vi "Vision 통합 수정필요.vi"() -> ()   [LabVIEW 2016]
uses:
  <vilib>/vision/Classification.llb/IMAQ Classifier Nearest Neighbor options.ctl
  <vilib>/vision/NI_Vision_Development_Module.lvlib
  <vilib>/ptbypt/NI_PtbyPt.lvlib
panel:
  in  "경로 설정":enum32{"주차", "유턴", "곡선", "동적"}(tab)
  in  "File Path (Particle Classification 1)":path=path "C:/Users/SeongHyeon/Desktop/[Github]_GPS Team/labview_program/작업중인 모든 Vi, dll파일 모음/전체프로그램/Sub Vi/Sensor/Vision Reference/주차.clf"
  in  "유턴File Path":path=path "C:/Users/SeongHyeon/Desktop/[Github]_GPS Team/labview_program/작업중인 모든 Vi, dll파일 모음/전체프로그램/Sub Vi/Sensor/Vision Reference/유턴2.clf"
  in  "곡선File Path 2":path=path "C:/Users/SeongHyeon/Desktop/[Github]_GPS Team/labview_program/작업중인 모든 Vi, dll파일 모음/전체프로그램/Sub Vi/Sensor/Vision Reference/곡선2.clf"
  in  "동적장애물File Path 4":path=path "C:/Users/SeongHyeon/Desktop/[Github]_GPS Team/labview_program/작업중인 모든 Vi, dll파일 모음/전체프로그램/Sub Vi/Sensor/Vision Reference/동적 장애물 Dark.clf"
  in  "Parameter 설정":enum32{"주차", "유턴", "곡선", "동적"}(tab)
  in  "주차 Paramaters":T2={"Preprocessing Options"={"Method"=-1, "Looking for"=1, "Threshold Range"={"Lower value"=0.0, "Upper value"=0.0}, "Threshold Limits"={"Lower value"=0.0, "Upper value"=0.0}, "Reject Border"=FALSE, "# of Erosions"=0, "Kernel Size"={"Lower value"=0, "Upper value"=0}, "Deviation Factor"=0.0}, "Nearest Neighbor Options"={"Method"=0, "Metric"=0, "k"=0}, "Particle Options"={"Scale Dependant"=FALSE, "Scale Factor"=0.0, "Symmetry Dependant"=FALSE, "Symmetry Factor"=0.0}} {"Preprocessing Options"."Deviation Factor" min=0.0; "Preprocessing Options"."Threshold Limits"."Upper value" format="%.2f"; "Preprocessing Options"."Threshold Limits"."Lower value" format="%.2f"; "Preprocessing Options"."Threshold Range"."Upper value" format="%.2f"; "Preprocessing Options"."Threshold Range"."Lower value" format="%.2f"; "Preprocessing Options"."# of Erosions" min=0; "Preprocessing Options"."Method" items=["Manual Threshold"=-1, "-"=-2, "Auto Threshold: Clustering"=0, "Auto Threshold: Entropy"=1, "Auto Threshold: Metric"=2, "Auto Threshold: Moments"=3, "Auto Threshold: Inter-class Variance"=4, "--"=-3, "Local Threshold: Niblack"=5, "Local Threshold: BG Correction"=6]; "Preprocessing Options"."Looking for" items=["Bright Objects", "Dark Objects"]; "Nearest Neighbor Options"."Method" items=["Nearest Neighbor", "K Nearest Neighbor", "Minimum Mean Distance"]; "Nearest Neighbor Options"."Metric" items=["Maximum", "Sum", "Euclidean"]; "Nearest Neighbor Options"."k" min=3}
  in  "유턴 Paramaters":T2={"Preprocessing Options"={"Method"=-1, "Looking for"=1, "Threshold Range"={"Lower value"=0.0, "Upper value"=0.0}, "Threshold Limits"={"Lower value"=0.0, "Upper value"=0.0}, "Reject Border"=FALSE, "# of Erosions"=0, "Kernel Size"={"Lower value"=0, "Upper value"=0}, "Deviation Factor"=0.0}, "Nearest Neighbor Options"={"Method"=0, "Metric"=0, "k"=0}, "Particle Options"={"Scale Dependant"=FALSE, "Scale Factor"=0.0, "Symmetry Dependant"=FALSE, "Symmetry Factor"=0.0}} {"Preprocessing Options"."Deviation Factor" min=0.0; "Preprocessing Options"."Threshold Limits"."Upper value" format="%.2f"; "Preprocessing Options"."Threshold Limits"."Lower value" format="%.2f"; "Preprocessing Options"."Threshold Range"."Upper value" format="%.2f"; "Preprocessing Options"."Threshold Range"."Lower value" format="%.2f"; "Preprocessing Options"."# of Erosions" min=0; "Preprocessing Options"."Method" items=["Manual Threshold"=-1, "-"=-2, "Auto Threshold: Clustering"=0, "Auto Threshold: Entropy"=1, "Auto Threshold: Metric"=2, "Auto Threshold: Moments"=3, "Auto Threshold: Inter-class Variance"=4, "--"=-3, "Local Threshold: Niblack"=5, "Local Threshold: BG Correction"=6]; "Preprocessing Options"."Looking for" items=["Bright Objects", "Dark Objects"]; "Nearest Neighbor Options"."Method" items=["Nearest Neighbor", "K Nearest Neighbor", "Minimum Mean Distance"]; "Nearest Neighbor Options"."Metric" items=["Maximum", "Sum", "Euclidean"]; "Nearest Neighbor Options"."k" min=3}
  in  "곡선 Paramaters":T2={"Preprocessing Options"={"Method"=-1, "Looking for"=1, "Threshold Range"={"Lower value"=0.0, "Upper value"=0.0}, "Threshold Limits"={"Lower value"=0.0, "Upper value"=0.0}, "Reject Border"=FALSE, "# of Erosions"=0, "Kernel Size"={"Lower value"=0, "Upper value"=0}, "Deviation Factor"=0.0}, "Nearest Neighbor Options"={"Method"=0, "Metric"=0, "k"=0}, "Particle Options"={"Scale Dependant"=FALSE, "Scale Factor"=0.0, "Symmetry Dependant"=FALSE, "Symmetry Factor"=0.0}} {"Preprocessing Options"."Deviation Factor" min=0.0; "Preprocessing Options"."Threshold Limits"."Upper value" format="%.2f"; "Preprocessing Options"."Threshold Limits"."Lower value" format="%.2f"; "Preprocessing Options"."Threshold Range"."Upper value" format="%.2f"; "Preprocessing Options"."Threshold Range"."Lower value" format="%.2f"; "Preprocessing Options"."# of Erosions" min=0; "Preprocessing Options"."Method" items=["Manual Threshold"=-1, "-"=-2, "Auto Threshold: Clustering"=0, "Auto Threshold: Entropy"=1, "Auto Threshold: Metric"=2, "Auto Threshold: Moments"=3, "Auto Threshold: Inter-class Variance"=4, "--"=-3, "Local Threshold: Niblack"=5, "Local Threshold: BG Correction"=6]; "Preprocessing Options"."Looking for" items=["Bright Objects", "Dark Objects"]; "Nearest Neighbor Options"."Method" items=["Nearest Neighbor", "K Nearest Neighbor", "Minimum Mean Distance"]; "Nearest Neighbor Options"."Metric" items=["Maximum", "Sum", "Euclidean"]; "Nearest Neighbor Options"."k" min=3}
  in  "동적 Paramaters":T2={"Preprocessing Options"={"Method"=-1, "Looking for"=1, "Threshold Range"={"Lower value"=0.0, "Upper value"=0.0}, "Threshold Limits"={"Lower value"=0.0, "Upper value"=0.0}, "Reject Border"=FALSE, "# of Erosions"=0, "Kernel Size"={"Lower value"=0, "Upper value"=0}, "Deviation Factor"=0.0}, "Nearest Neighbor Options"={"Method"=0, "Metric"=0, "k"=0}, "Particle Options"={"Scale Dependant"=FALSE, "Scale Factor"=0.0, "Symmetry Dependant"=FALSE, "Symmetry Factor"=0.0}} {"Preprocessing Options"."Deviation Factor" min=0.0; "Preprocessing Options"."Threshold Limits"."Upper value" format="%.2f"; "Preprocessing Options"."Threshold Limits"."Lower value" format="%.2f"; "Preprocessing Options"."Threshold Range"."Upper value" format="%.2f"; "Preprocessing Options"."Threshold Range"."Lower value" format="%.2f"; "Preprocessing Options"."# of Erosions" min=0; "Preprocessing Options"."Method" items=["Manual Threshold"=-1, "-"=-2, "Auto Threshold: Clustering"=0, "Auto Threshold: Entropy"=1, "Auto Threshold: Metric"=2, "Auto Threshold: Moments"=3, "Auto Threshold: Inter-class Variance"=4, "--"=-3, "Local Threshold: Niblack"=5, "Local Threshold: BG Correction"=6]; "Preprocessing Options"."Looking for" items=["Bright Objects", "Dark Objects"]; "Nearest Neighbor Options"."Method" items=["Nearest Neighbor", "K Nearest Neighbor", "Minimum Mean Distance"]; "Nearest Neighbor Options"."Metric" items=["Maximum", "Sum", "Euclidean"]; "Nearest Neighbor Options"."k" min=3}
  out "Image":T3(plugin-control)
  out "Identification Score":sgl
  out "주차냐":bool
  in  "ROI Descriptor (Particle Classification 1) 2":T4={"Global Rectangle"=[750, 250, 1250, 750], "Contours"=[{"ID"=enum."External", "Type"=3, "Coordinates"=[750, 399, 891, 593]}]} {"Contours"."Type" items=["No Selection", "Point", "Line", "Rectangle", "Oval", "Polygon", "Freehand Region", "Annulus", "Unused2", "Unused3", "Broken Line", "Freehand Line", "Rotated Rectangle"]}
  out "유턴이냐":bool
  out "횡단보도 거리":dbl[](array[numeric])
  out "곡선이냐":bool
  out "동적이냐":bool
  in  "Colors (Green)":u32[](array[colorbox])=[65280]
  out "Calibrated Results (Caliper 1)":sgl[][](array[numeric]) format="%.2f"
  out "Filtered image":T3(plugin-control)
  out "Original Image":T3(plugin-control)
  out "Original Image":T3(plugin-control)
  out "프레임 rate":dbl
  out "error out":errorcluster
  in  "이미지 형식":T5 items=["Grayscale (U8)", "Grayscale (I16)", "Grayscale (SGL)", "Complex (CSG)", "RGB (U32)", "HSL (U32)", "RGB (U64)", "Grayscale (U16)"]
  in  "Stop (F)":bool
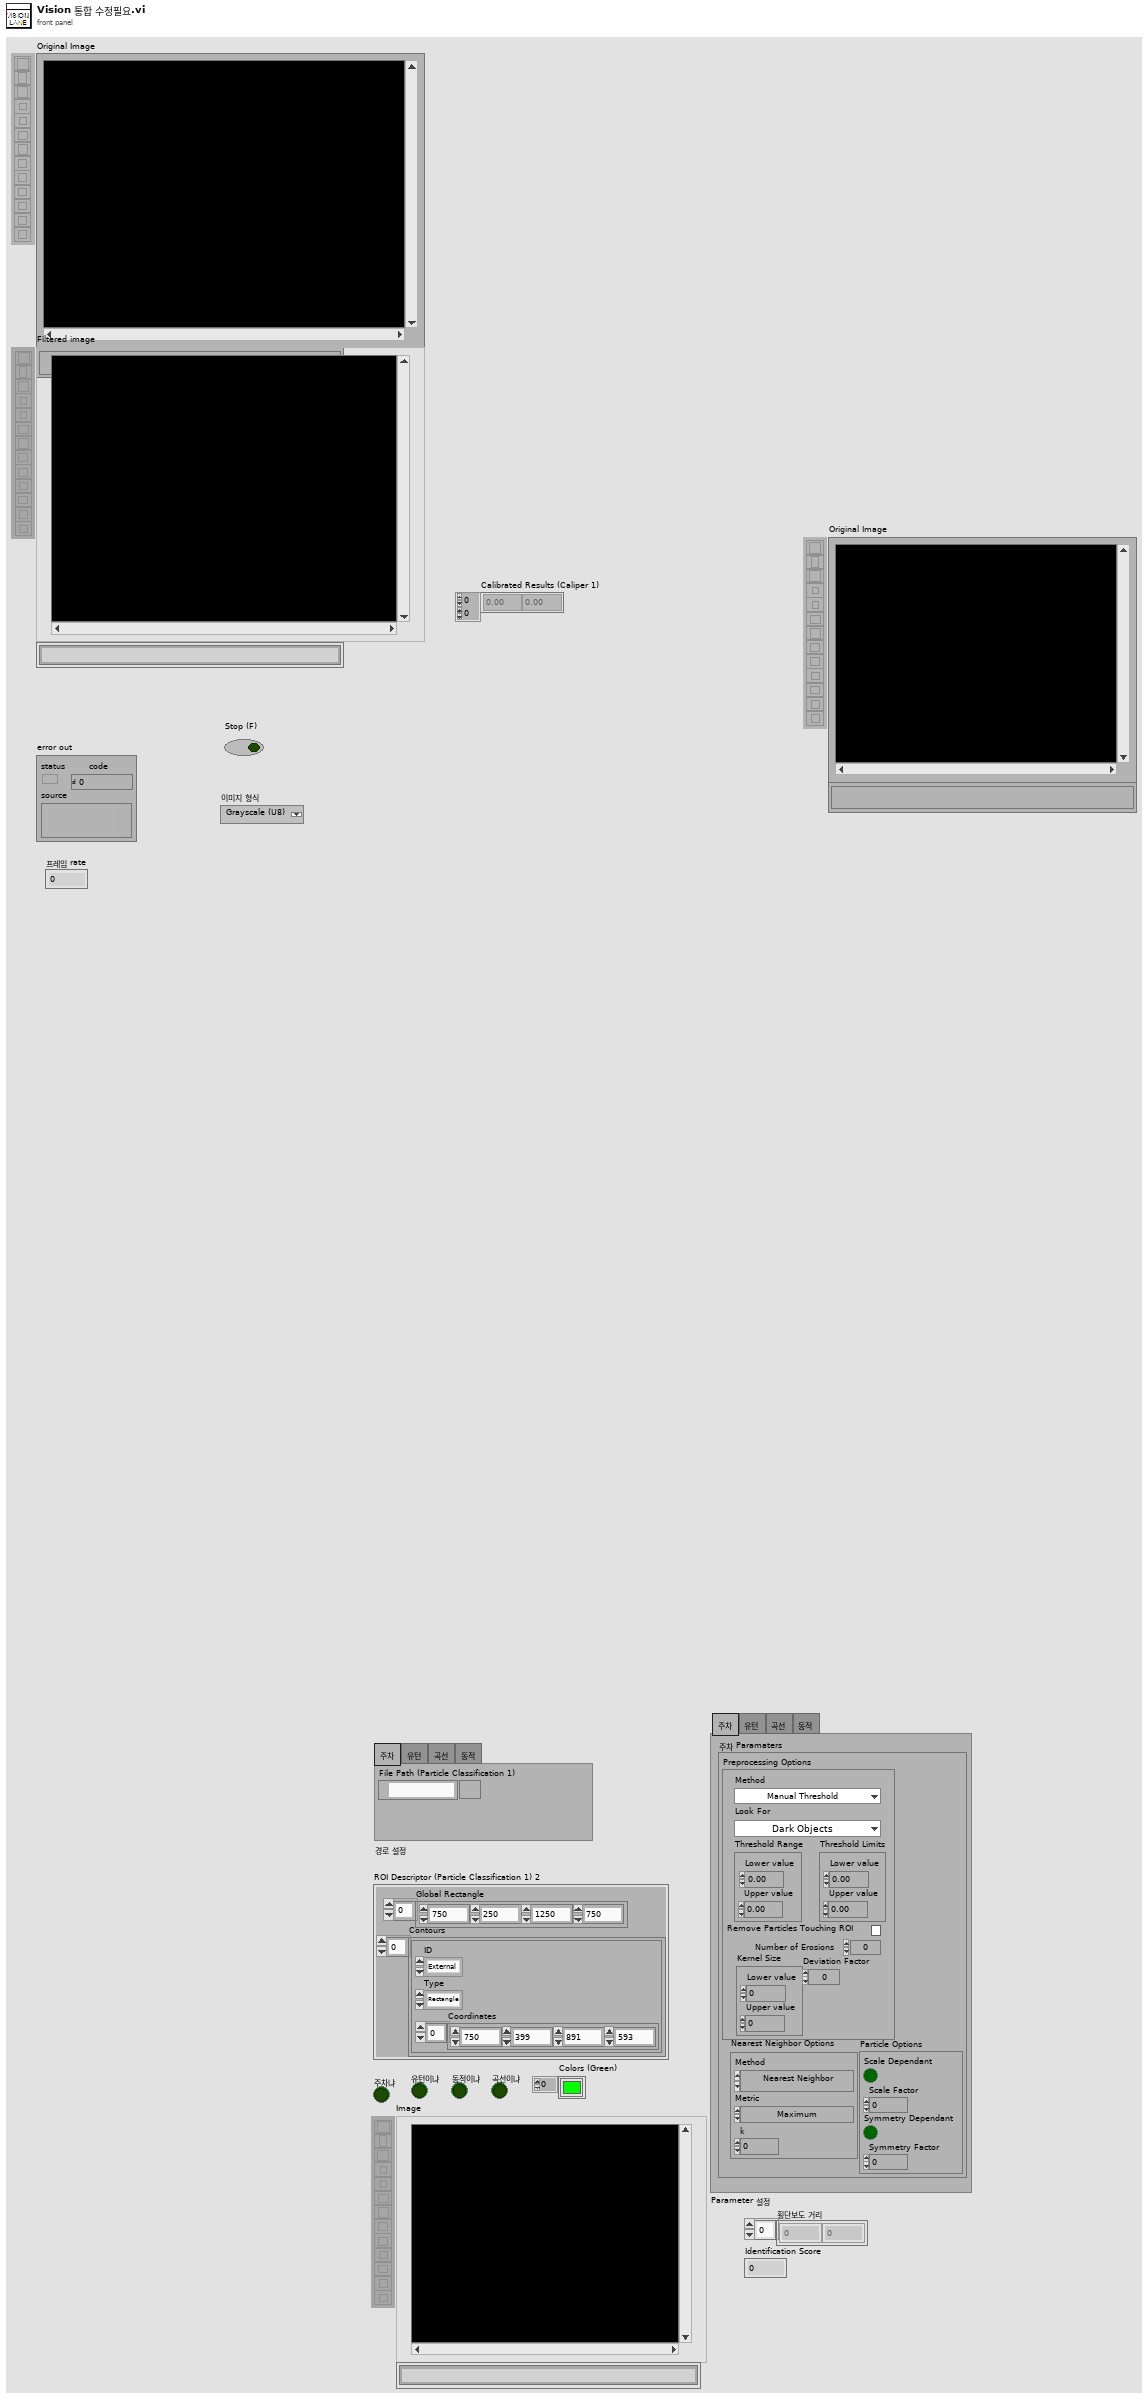
[diagram p1: front panel]
types:
  T1 = typedef "IMAQ Classifier Nearest Neighbor options.ctl" = cluster{"Method":i32, "Metric":i32, "k":i32}
  T2 = cluster{"Preprocessing Options":cluster{"Method":i32, "Looking for":i32, "Threshold Range":cluster{"Lower value":sgl, "Upper value":sgl}, "Threshold Limits":cluster{"Lower value":sgl, "Upper value":sgl}, "Reject Border":bool, "# of Erosions":i32, "Kernel Size":cluster{"Lower value":i32, "Upper value":i32}, "Deviation Factor":dbl}, "Nearest Neighbor Options":T1, "Particle Options":cluster{"Scale Dependant":bool, "Scale Factor":sgl, "Symmetry Dependant":bool, "Symmetry Factor":sgl}}
  T3 = typedef "IMAQ Image.ctl" = refnum<image>
  T4 = cluster{"Global Rectangle":i32[], "Contours":cluster{"ID":enum32{"External", "Internal"}, "Type":u32, "Coordinates":i32[]}[]}
  T5 = typedef "Image Type" = u32
  T6 = cluster{"Calibrated Results (Caliper 1)[0]":sgl, "Calibrated Results (Caliper 1)[1]":sgl, "Calibrated Results (Caliper 1)[2]":sgl, "Calibrated Results (Caliper 1)[3]":sgl, "Calibrated Results (Caliper 1)[4]":sgl, "Calibrated Results (Caliper 1)[5]":sgl, "Calibrated Results (Caliper 1)[6]":sgl, "Calibrated Results (Caliper 1)[7]":sgl, "Calibrated Results (Caliper 1)[8]":sgl}
  T7 = typedef "IMAQ Classifier Session.ctl" = refnum<k1>
  T8 = cluster{"Position":cluster{"x":sgl, "y":sgl}, "Angle":sgl, "Scale":sgl, "Score":sgl, "Bounding Box":cluster{"x":sgl, "y":sgl}[]}[]
  T9 = cluster{"Position":cluster{"x":sgl, "y":sgl}, "Angle":sgl, "Scale":sgl, "Score":sgl, "Bounding Box":cluster{"x":sgl, "y":sgl}[]}
  T10 = cluster{"Classification Score":sgl, "Identification Score":sgl}
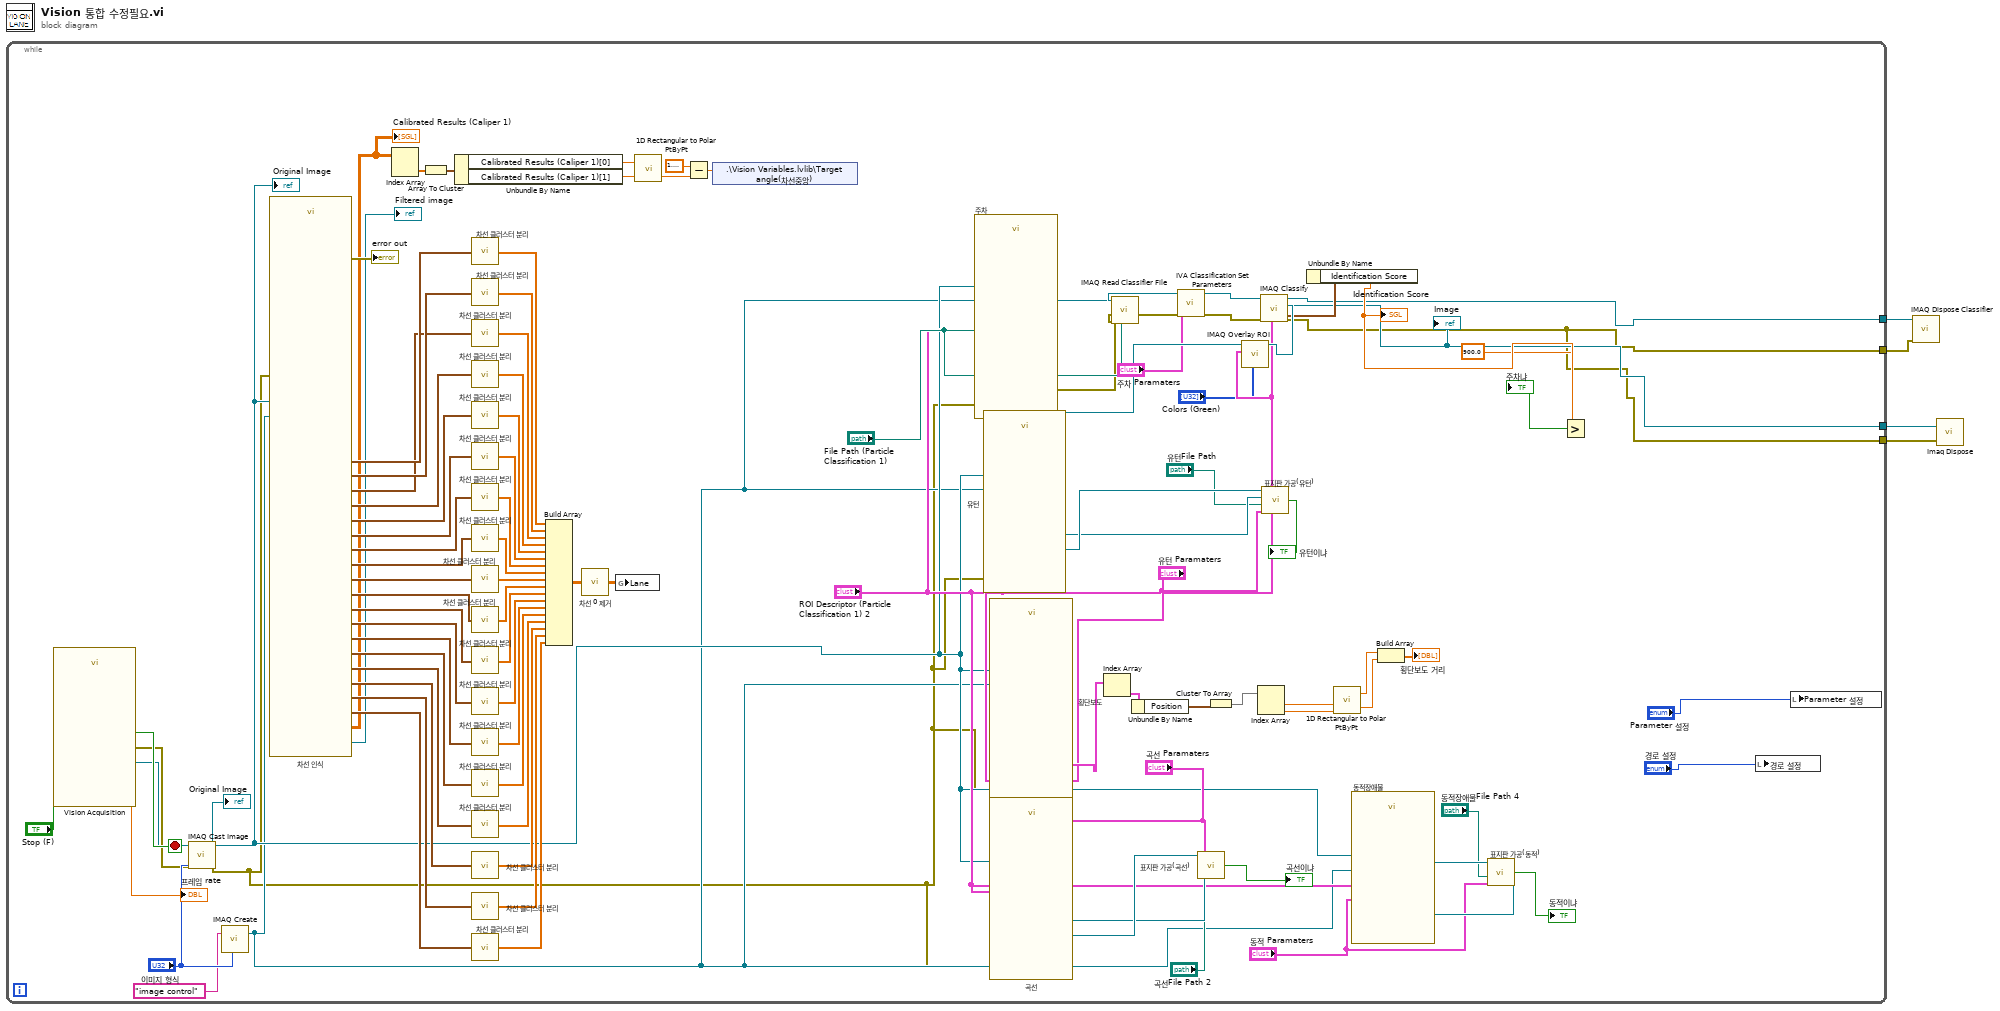
[diagram p0: block diagram]
diagram:
  n1 = while {
    tunnel: [w7] -> w4
    tunnel: [w5] -> w3
    tunnel: [w6] -> w2
    tunnel: [w5] -> w1
    stop <- w106 stop-if-true
    n2 = call "Vision Acquisition"("Stop (F)"="Stop (F)") -> ("Image Out"=w11:T3, "Frame Rate"=→"프레임 rate":dbl, "Stopped"=w106:bool, "error out"=w103:errorcluster)  [unwired: 23 in]
    "Original Image" <- w11
    n3 = call "IMAQ Cast Image"("Image Type"="이미지 형식", "error in (no error)"=w103, "Image Src"=w11) -> ("error out"=w8:errorcluster, "Image Dst Out"=w10:T3)  [unwired: 7 in]
    "Original Image" <- w10
    n4 = call "IMAQ Create"("Image Name"="image control", "Image Type"="이미지 형식") -> ("New Image"=w9:T3)  [unwired: 3 in, 1 out]
    n5 = call "차선 인식"("Image In"=w10, "Image Dst"=w9, "error in"=w8) -> ("Calibrated Results (Caliper 1)"=w63:sgl[][], "Edges Coordinates (calibrated) (Edge Detector 21)"=w81:cluster{"X":sgl, "Y":sgl}[], "Edges Coordinates (calibrated) (Edge Detector 20)"=w82:cluster{"X":sgl, "Y":sgl}[], "Edges Coordinates (calibrated) (Edge Detector 19)"=w83:cluster{"X":sgl, "Y":sgl}[], "Edges Coordinates (calibrated) (Edge Detector 18)"=w84:cluster{"X":sgl, "Y":sgl}[], "Edges Coordinates (calibrated) (Edge Detector 17)"=w85:cluster{"X":sgl, "Y":sgl}[], "Edges Coordinates (calibrated) (Edge Detector 16)"=w86:cluster{"X":sgl, "Y":sgl}[], "Edges Coordinates (calibrated) (Edge Detector 15)"=w87:cluster{"X":sgl, "Y":sgl}[], "Edges Coordinates (calibrated) (Edge Detector 13)"=w88:cluster{"X":sgl, "Y":sgl}[], "Edges Coordinates (calibrated) (Edge Detector 12)"=w89:cluster{"X":sgl, "Y":sgl}[], "Edges Coordinates (calibrated) (Edge Detector 11)"=w90:cluster{"X":sgl, "Y":sgl}[], "Edges Coordinates (calibrated) (Edge Detector 10)"=w91:cluster{"X":sgl, "Y":sgl}[], "Edges Coordinates (calibrated) (Edge Detector 8)"=w92:cluster{"X":sgl, "Y":sgl}[], "Edges Coordinates (calibrated) (Edge Detector 7)"=w93:cluster{"X":sgl, "Y":sgl}[], "Edges Coordinates (calibrated) (Edge Detector 5)"=w94:cluster{"X":sgl, "Y":sgl}[], "Image Out"=→"Filtered image":T3, "Edges Coordinates (calibrated) (Edge Detector 1)"=w100:cluster{"X":sgl, "Y":sgl}[], "Edges Coordinates (calibrated) (Edge Detector 2)"=w98:cluster{"X":sgl, "Y":sgl}[], "Edges Coordinates (calibrated) (Edge Detector 3)"=w96:cluster{"X":sgl, "Y":sgl}[], "Edges Coordinates (calibrated) (Edge Detector 4)"=w95:cluster{"X":sgl, "Y":sgl}[], "error out"=→"error out":errorcluster)  [unwired: 2 in, 2 out]
    "Calibrated Results (Caliper 1)" <- w63
    n6 = Index Array(array=w63) -> (element=w62:sgl[])  [unwired: 2 in]
    n7 = Array To Cluster(array=w62) -> (cluster=w61:T6)
    n8 = Unbundle By Name(w61) -> ("Calibrated Results (Caliper 1)[0]"=w60:sgl, "Calibrated Results (Caliper 1)[1]"=w59:sgl)
    n9 = call "차선 클러스터 분리.vi"("배열"=w100) -> ("R, Theta"=w99:dbl[])
    n10 = call "차선 클러스터 분리.vi"("배열"=w98) -> ("R, Theta"=w97:dbl[])
    n11 = call "차선 클러스터 분리.vi"("배열"=w96) -> ("R, Theta"=w80:dbl[])
    n12 = call "차선 클러스터 분리.vi"("배열"=w95) -> ("R, Theta"=w79:dbl[])
    n13 = call "차선 클러스터 분리.vi"("배열"=w94) -> ("R, Theta"=w78:dbl[])
    n14 = call "차선 클러스터 분리.vi"("배열"=w93) -> ("R, Theta"=w77:dbl[])
    n15 = call "차선 클러스터 분리.vi"("배열"=w92) -> ("R, Theta"=w76:dbl[])
    n16 = call "차선 클러스터 분리.vi"("배열"=w91) -> ("R, Theta"=w75:dbl[])
    n17 = call "차선 클러스터 분리.vi"("배열"=w90) -> ("R, Theta"=w74:dbl[])
    n18 = call "차선 클러스터 분리.vi"("배열"=w89) -> ("R, Theta"=w73:dbl[])
    n19 = call "차선 클러스터 분리.vi"("배열"=w88) -> ("R, Theta"=w72:dbl[])
    n20 = call "차선 클러스터 분리.vi"("배열"=w87) -> ("R, Theta"=w71:dbl[])
    n21 = call "차선 클러스터 분리.vi"("배열"=w86) -> ("R, Theta"=w70:dbl[])
    n22 = call "차선 클러스터 분리.vi"("배열"=w85) -> ("R, Theta"=w69:dbl[])
    n23 = call "차선 클러스터 분리.vi"("배열"=w84) -> ("R, Theta"=w67:dbl[])
    n24 = call "차선 클러스터 분리.vi"("배열"=w83) -> ("R, Theta"=w66:dbl[])
    n25 = call "차선 클러스터 분리.vi"("배열"=w82) -> ("R, Theta"=w65:dbl[])
    n26 = call "차선 클러스터 분리.vi"("배열"=w81) -> ("R, Theta"=w64:dbl[])
    n27 = Build Array(w99, w97, w80, w79, w78, w77, w76, w75, w74, w73, w72, w71, w70, w69, w67, w66, w65, w64) -> (w56:dbl[][])
    n28 = call "차선 0 제거.vi"("추가된 배열"=w56) -> ("제거된 배열"=w55:dbl[][])
    n29 = global write "[GV]_Vision Lane.vi" "Lane"(w55) -> ()
    n30 = call <vilib>:"1D Rectangular to Polar PtByPt.vi"("y"=w59, "x"=w60) -> ("phase"=w57:dbl)  [unwired: 1 out]
    n31 = Subtract(x=1.5707963267948966, y=w57) -> (x-y=w54:dbl)
    n32 = shared-variable ".\\Vision Variables.lvlib\\Target angle(차선중앙)"(w54) -> ()  [unwired: 1 in, 1 out]
    n33 = call "주차"("Image In"=w10, "Image Dst"=w9, "ROI Descriptor (Particle Classification 1)"="ROI Descriptor (Particle Classification 1) 2", "File Path (Particle Classification 1)"="File Path (Particle Classification 1)", "error in"=w8) -> ("Image Out"=w42:T3, "Classifier Session (Particle Classification 1)"=w40:T7, "error out"=w39:errorcluster)  [unwired: 20 in]
    n34 = call "유턴"("Image In"=w10, "Image Dst"=w9, "ROI Descriptor (Particle Classification 1)"="ROI Descriptor (Particle Classification 1) 2", "Parameters (Particle Classification 1)"="유턴 Paramaters", "error in"=w8) -> ("Image Out"=w37:T3, "Classifier Session (Particle Classification 1)"=w36:T7)  [unwired: 20 in, 1 out]
    n35 = call "횡단보도"("Image In"=w10, "Image Dst"=w9, "error in"=w8) -> ("Calibrated Matches (Pattern Matching 1)"=w31:T8)  [unwired: 22 in, 2 out]
    n36 = call "곡선"("Image In"=w10, "ROI Descriptor (Particle Classification 1)"="ROI Descriptor (Particle Classification 1) 2", "Parameters (Particle Classification 1)"="곡선 Paramaters", "error in"=w8) -> ("Image Out"=w33:T3, "Classifier Session (Particle Classification 1)"=w22:T7)  [unwired: 21 in, 1 out]
    n37 = Index Array(array=w31) -> (element=w30:T9)  [unwired: 1 in]
    n38 = call "IMAQ Read Classifier File"("File Path"="File Path (Particle Classification 1)", "error in (no error)"=w39, "Classifier Session (optional)"=w40) -> ("error out"=w48:errorcluster, "Classifier Session"=w49:T7)  [unwired: 4 in, 3 out]
    n39 = Unbundle By Name(w30) -> ("Position"=w29:cluster{"x":sgl, "y":sgl})
    n40 = call <vilib>:"IVA Classification Set Parameters.vi"("error in"=w48, "Paramaters"="주차 Paramaters", "Classifier Session In"=w49) -> ("error out"=w47:errorcluster, "Classifier Session Out"=w43:T7)  [unwired: 7 out]
    n41 = call "표지판 가공(곡선).vi"("Paramaters"="곡선 Paramaters", "File Path"="곡선File Path 2", "Classifier Session (optional)"=w22, "Image 2"=w33) -> ("주차냐"=→"곡선이냐":bool)
    n42 = Cluster To Array(cluster=w29) -> (array=w28:sgl[])
    n43 = call "IMAQ Overlay ROI"("Colors (Green)"="Colors (Green)", "ROI Descriptor"="ROI Descriptor (Particle Classification 1) 2", "Image"=w42) -> ("Image Out"=w51:T3)  [unwired: 7 in, 1 out]
    n44 = Index Array(array=w28) -> (element #1=w27:sgl, element #2=w26:sgl)  [unwired: 2 in]
    n45 = call "IMAQ Classify"("ROI Descriptor"="ROI Descriptor (Particle Classification 1) 2", "error in (no error)"=w47, "Image"=w51, "Classifier Session"=w43) -> ("error out"=w5:errorcluster, "Image (dup)"=w7:T3, "Classifier Session (dup)"=w6:T7, "Scores"=w50:T10)  [unwired: 2 in, 2 out]
    "Image" <- w7
    n46 = call "표지판 가공(유턴).vi"("Paramaters"="유턴 Paramaters", "File Path"="유턴File Path", "Classifier Session (optional)"=w36, "Image 2"=w37) -> ("주차냐"=→"유턴이냐":bool)
    n47 = Unbundle By Name(w50) -> ("Identification Score"=w46:sgl)
    "Identification Score" <- w46
    n48 = call <vilib>:"1D Rectangular to Polar PtByPt.vi"("y"=w26, "x"=w27) -> ("phase"=w24:dbl, "magnitude"=w25:dbl)
    n49 = call "동적장애물"("Image In"=w10, "Image Dst"=w9, "ROI Descriptor (Particle Classification 1)"="ROI Descriptor (Particle Classification 1) 2", "Parameters (Particle Classification 1)"="동적 Paramaters") -> ("Image Out"=w20:T3, "Classifier Session (Particle Classification 1)"=w19:T7)  [unwired: 21 in, 1 out]
    n50 = Build Array(w25, w24) -> (→"횡단보도 거리":dbl[])
    n51 = call "표지판 가공(동적).vi"("Paramaters"="동적 Paramaters", "File Path"="동적장애물File Path 4", "Classifier Session (optional)"=w19, "Image 2"=w20) -> ("주차냐"=→"동적이냐":bool)
    n52 = Greater?(x=w46, y=sgl 900.0) -> (0:→"주차냐":bool)
    n53 = local write "경로 설정"("경로 설정") -> ()
    n54 = local write "Parameter 설정"("Parameter 설정") -> ()
  }
  n55 = call "IMAQ Dispose Classifier"("error in (no error)"=w1, "Classifier Session"=w2) -> ()  [unwired: 9 in, 1 out]
  n56 = call "Imaq Dispose"("Image"=w4, "error in (no error)"=w3) -> ()  [unwired: 4 in, 1 out]
